vi "Cubic Function.vi"(1 "x":refnum<class "Dual.lvclass">) -> (0 "f(x)":refnum<class "Dual.lvclass">)   [LabVIEW 2020, in "Examples.lvlib"]
doc: "f(x) = (x/2)^2 * (x-3)"
uses:
  classes/Dual/Dual.lvclass
  classes/Dual/Dual.lvclass/Dual.ctl
  0eb4dda3-5bd7-4847-9a30-514c0416222e.vi
  7805c8b1-a590-4d51-98fb-eb1755892a98.vi
  2339b2d4-4176-426a-a400-f0798d2c3531.vi
  1dc40f4b-cd1a-4eea-ab3f-554bb7f0e0e1.vi
  0eb4dda3-5bd7-4847-9a30-514c0416222e.vi/24a95623-6a1f-44d7-8ceb-f913d85de021.vi
  0eb4dda3-5bd7-4847-9a30-514c0416222e.vi/5c488bfd-3ecc-489d-aaaa-34957662e42e.vi
  classes/Dual/Read a and b.vi
  classes/Dual/Write a and b.vi
  7805c8b1-a590-4d51-98fb-eb1755892a98.vi/957074e8-cc3b-4647-8ff1-d975a744cd4e.vi
  2339b2d4-4176-426a-a400-f0798d2c3531.vi/968883c3-f1f3-473a-bfc5-8cde3e5b01f7.vi
  2339b2d4-4176-426a-a400-f0798d2c3531.vi/bec82738-76c0-439a-a1c7-54fdd631a6e8.vi
  1dc40f4b-cd1a-4eea-ab3f-554bb7f0e0e1.vi/b6499733-2759-4852-aa6b-3ec1516ef704.vi
  1dc40f4b-cd1a-4eea-ab3f-554bb7f0e0e1.vi/ce7907ec-4dc6-4618-8708-ad667a8e3a23.vi
  0eb4dda3-5bd7-4847-9a30-514c0416222e.vi/5c488bfd-3ecc-489d-aaaa-34957662e42e.vi/5957e011-cf56-4527-b6ed-13c3a4ca997b.vi
  classes/Dual/Write a.vi
  2339b2d4-4176-426a-a400-f0798d2c3531.vi/bec82738-76c0-439a-a1c7-54fdd631a6e8.vi/5957e011-cf56-4527-b6ed-13c3a4ca997b.vi
  Examples.lvlib
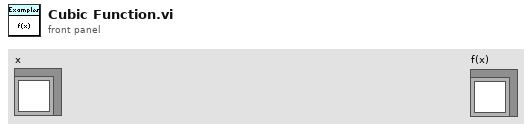
[diagram p1: front panel]
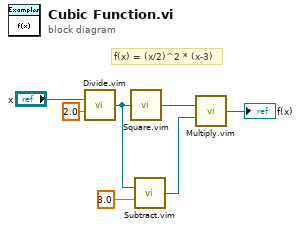
[diagram p0: block diagram]
diagram:
  # "f(x) = (x/2)^2 * (x-3)"
  n1 = call "Divide.vim"("x"="x", "y"=2.0 ("a")) -> ("x/y"=w3:refnum<class "Dual.lvclass">)  [unwired: 13 in]
  n2 = call "Square.vim"("x"=w3) -> ("x^2"=w7:refnum<class "Dual.lvclass">)
  n3 = call "Subtract.vim"("x"=w3, "y"=3.0 ("a")) -> ("x - y"=w2:refnum<class "Dual.lvclass">)  [unwired: 13 in]
  n4 = call "Multiply.vim"("x"=w7, "y"=w2) -> ("x * y"=→"f(x)":refnum<class "Dual.lvclass">)  [unwired: 13 in]
